vi "CRYCheck Channel Repeat.vi"(11 "Selected channel Info":T1[](array[typedef]) {"Coupling" items=["Default"=-1, "RSE"=10083, "NRSE"=10078, "Differential"=10106, "Pseudodifferential"=12529]; "term config" items=["Default"=-1, "RSE"=10083, "NRSE"=10078, "Differential"=10106, "Pseudodifferential"=12529]; "Anti-aliasing Factor (%fs)" format="%.2f"}) -> (3 "Run flag":bool)   [LabVIEW 2013]
uses:
  Typedef Control/CRYHardware Channel Info.ctl
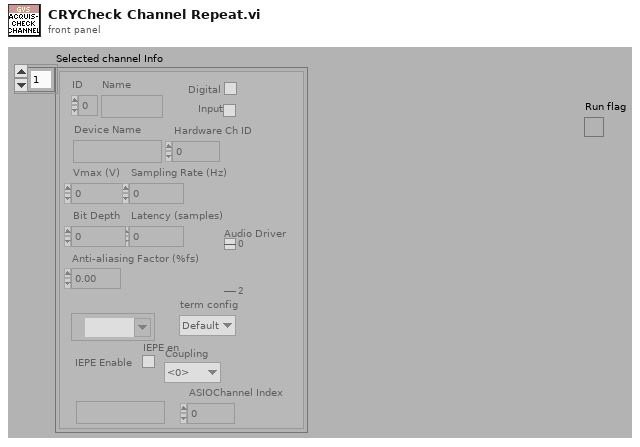
[diagram p1: front panel]
types:
  T1 = typedef "CRYHardware Channel Info.ctl" = cluster{"ID":i32, "Name":string, "Digital":bool, "Input":bool, "Device Name":string, "Hardware Ch ID":u8, "Vmax (V)":dbl, "Latency (samples)":dbl, "Sampling Rate (Hz)":u32, "Bit Depth":u32, "Anti-aliasing Factor (%fs)":sgl, "DAQmx Channel":tag, "term config":i32, "Coupling":i32, "IEPE en":bool, "ASIOChannel Name":string, "Audio Driver":u16, "ASIOChannel Index":u8}
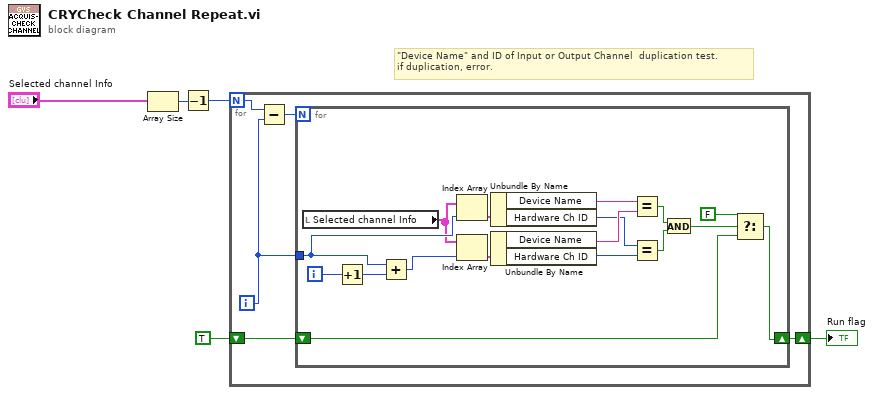
[diagram p0: block diagram]
diagram:
  # "\"Device Name\" and ID of Input or Output Channel  duplication test.\nif duplication, error."
  n1 = Array Size(array="Selected channel Info") -> (size(s)=w4:i32)
  n2 = Decrement(x=w4) -> (x-1=w5:i32)
  n3 = for {
    N: w5 -> [w10]
    shift-right: [w7] -> w1
    shift-left: TRUE ("Run flag") -> [w6]
    i -> [w8]
    n4 = Subtract(x=w10, y=w8) -> (x-y=w9:i32)
    n5 = for {
      N: w9 -> [_]
      tunnel: w8 -> [w22]
      shift-right: [w11] -> w7
      shift-left: w6 -> [w12]
      i -> [w25]
      n6 = local read "Selected channel Info"() -> (w19:T1[])
      n7 = Increment(x=w25) -> (x+1=w23:i32)
      n8 = Add(x=w22, y=w23) -> (x+y=w26:i32)
      n9 = Index Array(array=w19, index=w22) -> (element=w24:T1)
      n10 = Index Array(array=w19, index=w26) -> (element=w27:T1)
      n11 = Unbundle By Name(w24) -> ("Device Name"=w15:string, "Hardware Ch ID"=w16:u8)
      n12 = Unbundle By Name(w27) -> ("Device Name"=w17:string, "Hardware Ch ID"=w18:u8)
      n13 = Equal?(x=w15, y=w17) -> (x = y?=w21:bool)
      n14 = Equal?(x=w16, y=w18) -> (x = y?=w20:bool)
      n15 = And(x=w21, y=w20) -> (x .and. y?=w14:bool)
      n16 = Select(t=FALSE ("Run flag"), s=w14, f=w12) -> (s? t:f=w11:bool)
    }
  }
  "Run flag" <- w1
